vi "RemoveGear Get.vi"(1 "gear in":cluster{"a in":bool, "b in ":bool}) -> (0 "gear out":cluster{"a out":bool, "b out ":bool})   [LabVIEW 2016]
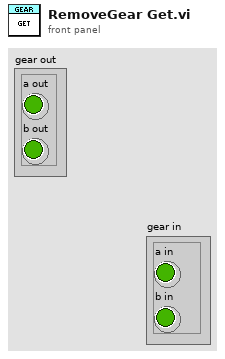
[diagram p1: front panel]
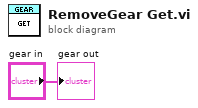
[diagram p0: block diagram]
diagram:
  "gear out" <- "gear in"
